vi "GetControlValuesDisplayName.vi"(11 "Name in":string) -> (2 "Display Name":string, 3 "Name":string)   [LabVIEW 2019]
uses:
  <vilib>/regexp/Match Regular Expression.xnode
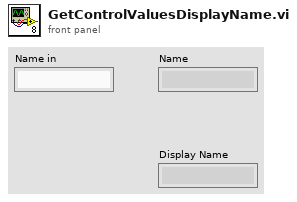
[diagram p1: front panel]
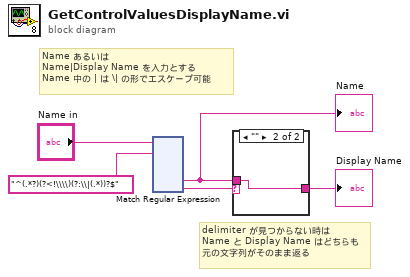
[diagram p0: block diagram]
diagram:
  # "Name あるいは\nName|Display Name を入力とする\nName 中の | は \\| の形でエスケープ可能"
  # "delimiter が見つからない時は\nName と Display Name はどちらも\n元の文字列がそのまま返る"
  n1 = xnode "Match Regular Expression"("input string"="Name in", "regular expression"="^(.*?)(?<!\\\\)(?:\\|(.*))?$") -> ("submatch 1"=w3:string, "submatch 2"=w1:string)  [unwired: 4 in, 5 out]
  "Name" <- w3
  n2 = case shown="\"\"" w1 {
    selector: w1 -> [w6 _]
    tunnel: w3 -> [_ w7]
    tunnel: [w6 w7] -> w2
    frame Default {
    }
    frame "" {
    }
  }
  "Display Name" <- w2
